vi "AlliGator Download Installer.vi"(6 "Show File?":bool, 8 "Error In":errorcluster, 9 "timeout (10000)":i32=10000, 10 "Dest Folder":path=path "C:/", 11 "URL":string) -> (0 "Error Out":errorcluster, 1 "body":string, 2 "headers":string, 3 "File Path":path)   [LabVIEW 2021, in "AlliGator GUI.lvlib"]
doc: "Downloads AlliGator installer from the provided URL."
uses:
  AlliGator GUI.lvlib
  <vilib>/httpClient/LabVIEWHTTPClient.lvlib
  Web/Web.lvlib
panel:
  # "see the AlliGator License on the block diagram (Ctrl+E or Window:Show Block Diagram)"
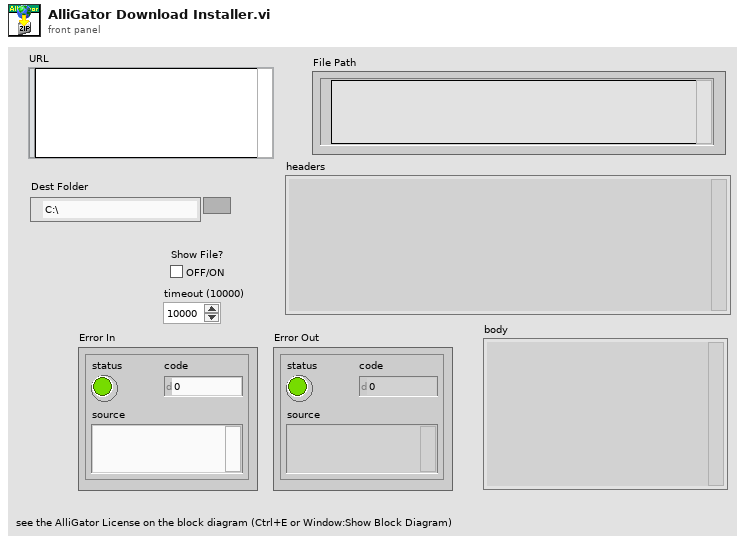
[diagram p1: front panel]
types:
  T1 = typedef "LabVIEWHTTPClient.lvlib/ClientHandle.ctl" = refnum<k1>
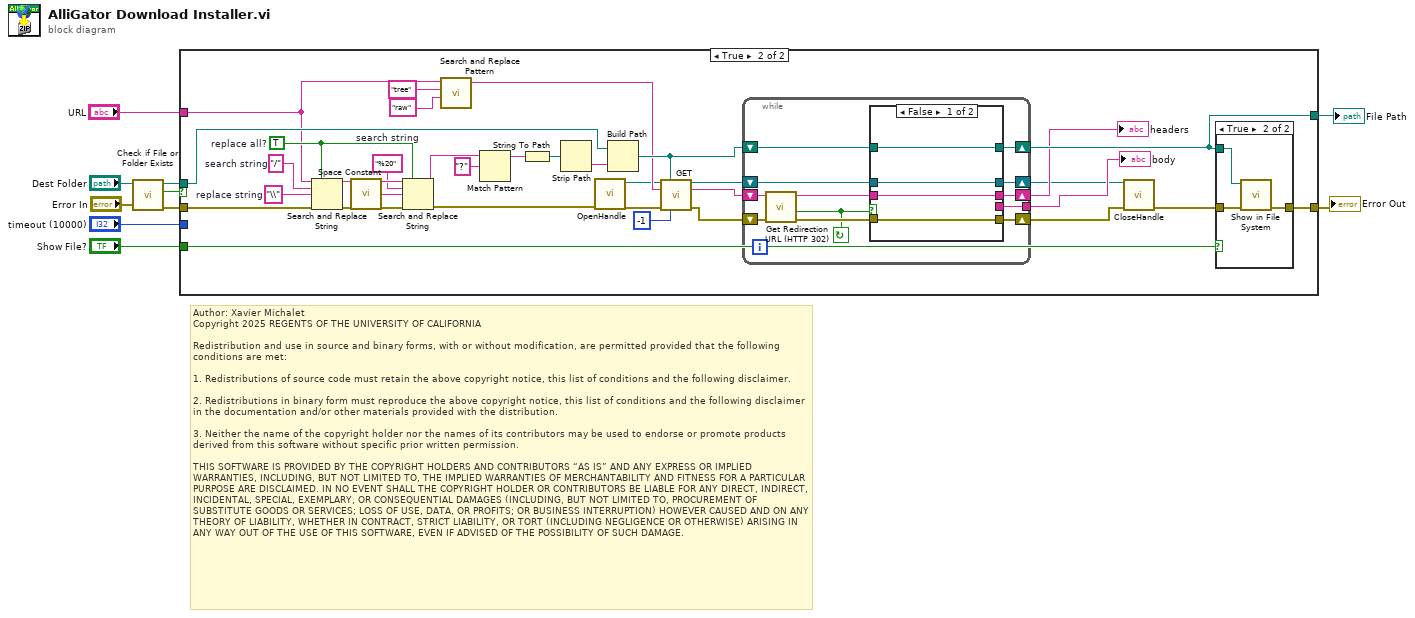
[diagram p0: block diagram]
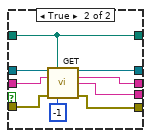
[diagram p3: hidden frame]
diagram:
  # "Author: Xavier Michalet\nCopyright 2025 REGENTS OF THE UNIVERSITY OF CALIFORNIA\n\nRedistribution and use in source and binary forms, with or without modification, are permitted provided that the following conditions are met:\n\n1. Redistributions of source code must retain the above copyright notice, this list of conditions and the following disclaimer.\n\n2. Redistributions in binary form must reproduce the above copyright notice, this list of conditions and the following disclaimer in the documentation and/or other materials provided with the distribution.\n\n3. Neither the name of the copyright holder nor the names of its contributors may be used to endorse or promote products derived from this software without specific prior written permission.\n\nTHIS SOFTWARE IS PROVIDED BY THE COPYRIGHT HOLDERS AND CONTRIBUTORS “AS IS” AND ANY EXPRESS OR IMPLIED WARRANTIES, INCLUDING, BUT NOT LIMITED TO, THE IMPLIED WARRANTIES OF MERCHANTABILITY AND FITNESS FOR A PARTICULAR PURPOSE ARE DISCLAIMED. IN NO EVENT SHALL THE COPYRIGHT HOLDER OR CONTRIBUTORS BE LIABLE FOR ANY DIRECT, INDIRECT, INCIDENTAL, SPECIAL, EXEMPLARY, OR CONSEQUENTIAL DAMAGES (INCLUDING, BUT NOT LIMITED TO, PROCUREMENT OF SUBSTITUTE GOODS OR SERVICES; LOSS OF USE, DATA, OR PROFITS; OR BUSINESS INTERRUPTION) HOWEVER CAUSED AND ON ANY THEORY OF LIABILITY, WHETHER IN CONTRACT, STRICT LIABILITY, OR TORT (INCLUDING NEGLIGENCE OR OTHERWISE) ARISING IN ANY WAY OUT OF THE USE OF THIS SOFTWARE, EVEN IF ADVISED OF THE POSSIBILITY OF SUCH DAMAGE."
  n1 = call <vilib>:"Check if File or Folder Exists.vi"("error in (no error)"="Error In", "path"="Dest Folder") -> ("error out"=w8:errorcluster, "file or folder exists?"=w5:bool, "dup path"=w7:path)  [unwired: 7 in]
  n2 = case shown="True" w5 {
    tunnel: "URL" -> [_ w19]
    tunnel: w8 -> [w11 w41]
    tunnel: w7 -> [_ w38]
    tunnel: [w11 w40] -> w2
    tunnel: "Show File?" -> [_ w39]
    tunnel: "timeout (10000)" -> [_ _]
    tunnel: [_ w27] -> w1
    frame False {
    }
    frame True {
      w31 = "%20"  # search string
      w32 = TRUE  # replace all?
      w44 = "\\"  # replace string
      w45 = "/"  # search string
      n3 = Search and Replace String(replace all?=w32, input string=w19, search string=w45, replace string=w44, error in=w41) -> (result string=w34:string, error out=w35:errorcluster)  [unwired: 3 in, 2 out]
      n4 = call <vilib>:"Space Constant.vi"() -> ("String"=w30:string)
      n5 = Search and Replace String(replace all?=w32, input string=w34, search string=w31, replace string=w30, error in=w35) -> (result string=w33:string, error out=w16:errorcluster)  [unwired: 3 in, 2 out]
      n6 = call <vilib>:"Search and Replace Pattern.vi"("string"=w19, "regular expression (\"\")"="tree" ("regular expression (\"\")"), "replace string (\"\")"="raw" ("replace string (\"\")")) -> ("result string"=w20:string)  [unwired: 2 in, 1 out]
      n7 = Match Pattern(string=w33, regular expression="?") -> (before substring=w36:string)  [unwired: 1 in, 3 out]
      n8 = String To Path(string=w36) -> (path=w43:path)
      n9 = Strip Path(path=w43) -> (name=w42:string)  [unwired: 1 out]
      n10 = call <vilib>:"OpenHandle.vi"("error in (no error)"=w16) -> ("client handle out"=w14:T1, "error out"=w15:errorcluster)  [unwired: 13 in]
      n11 = Build Path(base path=w38, name or relative path=w42) -> (appended path=w23:path)
      n12 = call <vilib>:"GET.vi"("client handle"=w14, "output file"=w23, "url"=w20, "error in (no error)"=w15, "timeout (10000)"=-1) -> ("client handle out"=w28:T1, "headers"=w22:string, "error out"=w29:errorcluster)  [unwired: 7 in, 1 out]
      n13 = while {
        shift-right: [w51] -> w26
        shift-left: w29 -> [w57]
        shift-right: [w47] -> w24
        shift-left: w22 -> [w53]
        shift-right: [w55] -> w12
        shift-left: w28 -> [w56]
        shift-right: [w50] -> w27
        shift-left: w23 -> [w52]
        tunnel: [w49] -> w25
        stop <- w46 continue-if-true
        n14 = call "Get Redirection URL (HTTP 302).vi"("error in (no error)"=w57, "HTTP GET Header"=w53) -> ("error out"=w54:errorcluster, "redirection"=w46:bool, "Redirection URL"=w48:string)  [unwired: 7 in]
        n15 = case shown="False" w46 {
          tunnel: w56 -> [w61 w70]
          tunnel: [w61 w69] -> w55
          tunnel: w54 -> [w58 w68]
          tunnel: w48 -> [w60 w67]
          tunnel: [w60 w64] -> w47
          tunnel: w52 -> [w59 w65]
          tunnel: [w58 w66] -> w51
          tunnel: [w59 w65] -> w50
          tunnel: [_ w63] -> w49
          frame False {
          }
          frame True {
            n16 = call <vilib>:"GET.vi"("client handle"=w70, "output file"=w65, "url"=w67, "error in (no error)"=w68, "timeout (10000)"=-1) -> ("client handle out"=w69:T1, "headers"=w64:string, "body"=w63:string, "error out"=w66:errorcluster)  [unwired: 7 in]
          }
        }
      }
      "headers" <- w24
      "body" <- w25
      n17 = call <vilib>:"CloseHandle.vi"("client handle"=w12, "error in (no error)"=w26) -> ("error out"=w21:errorcluster)  [unwired: 13 in]
      n18 = case shown="True" w39 {
        tunnel: w27 -> [_ w74]
        tunnel: w21 -> [w71 w73]
        tunnel: [w71 w72] -> w40
        frame False {
        }
        frame True {
          n19 = call <vilib>:"Show in File System.vi"("error in (no error)"=w73, "file or directory path"=w74) -> ("error out"=w72:errorcluster)  [unwired: 9 in]
        }
      }
    }
  }
  "Error Out" <- w2
  "File Path" <- w1
